vi "password.vi"() -> (0 "correct":bool)   [LabVIEW 2019]
uses:
  LLB/Commonly VI/Main Glb.vi
  <vilib>/Utility/xml.llb/Read From XML File(string).vi
  <vilib>/Utility/xml.llb/Write to XML File(string).vi
  Function/RobotCtrl Folder/Global/Robot_LinkData.vi
  LLB/Commonly VI.lvlib
panel:
  in  "Tab Control":enum32{"Page 1", "Page 2"}(tab)
  in  "1":bool
  in  "2":bool
  in  "3":bool
  in  "4":bool
  in  "5":bool
  in  "6":bool
  in  "7":bool
  in  "8":bool
  in  "9":bool
  in  "0":bool
  in  "String":string
  in  "check":bool
  in  "Cancel Button":bool
  in  "Seek Back Button":bool
  in  "Settings Button":bool
  in  "Stop Button":bool
  out "password":string
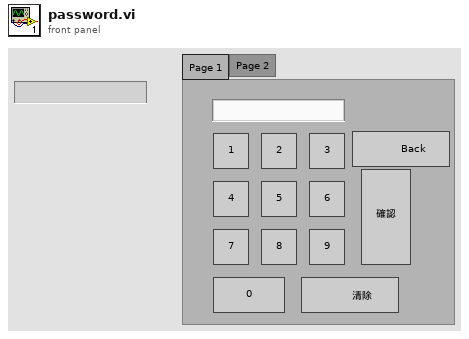
[diagram p1: front panel]
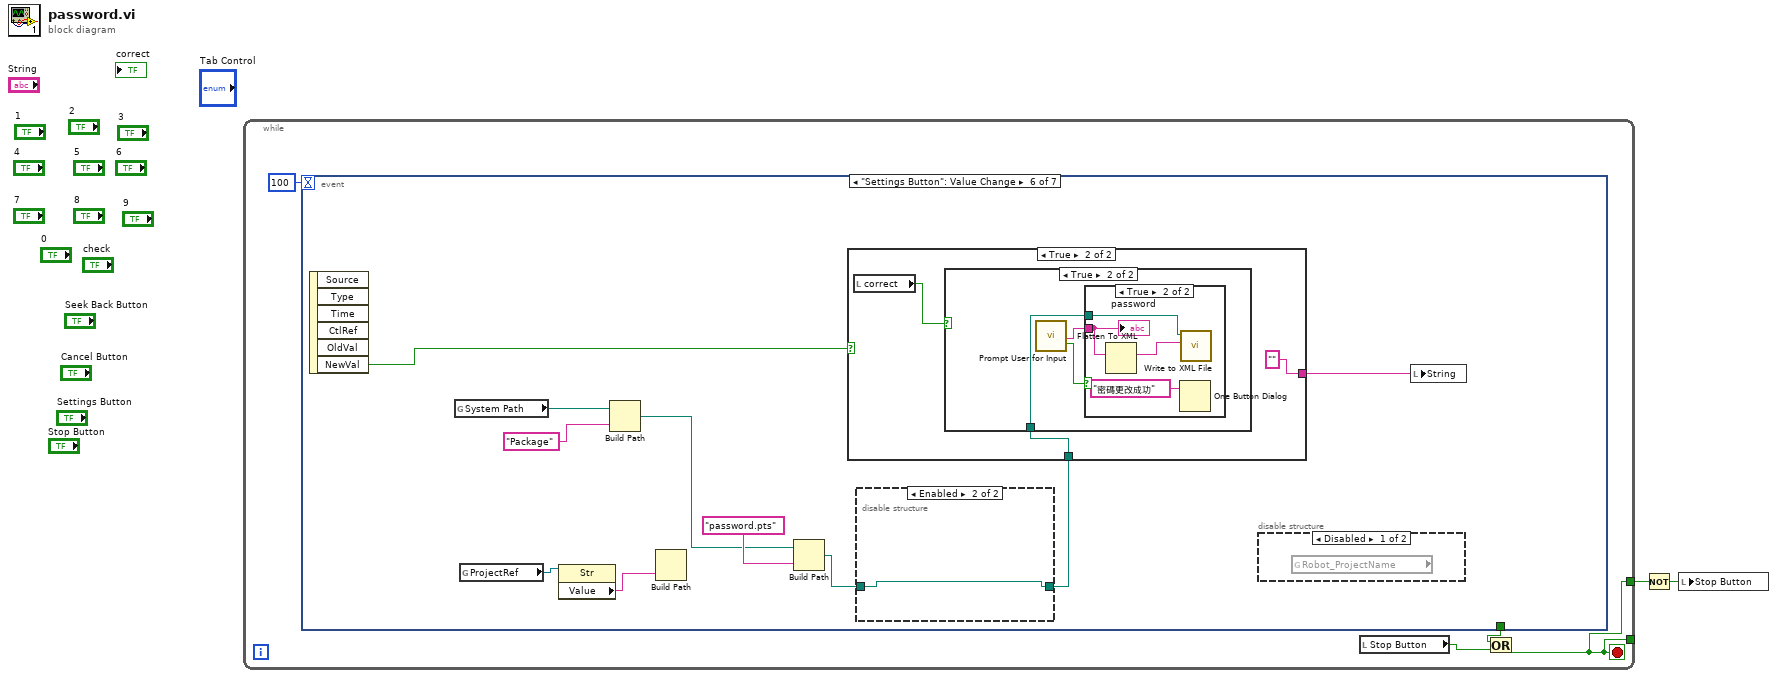
[diagram p0: block diagram]
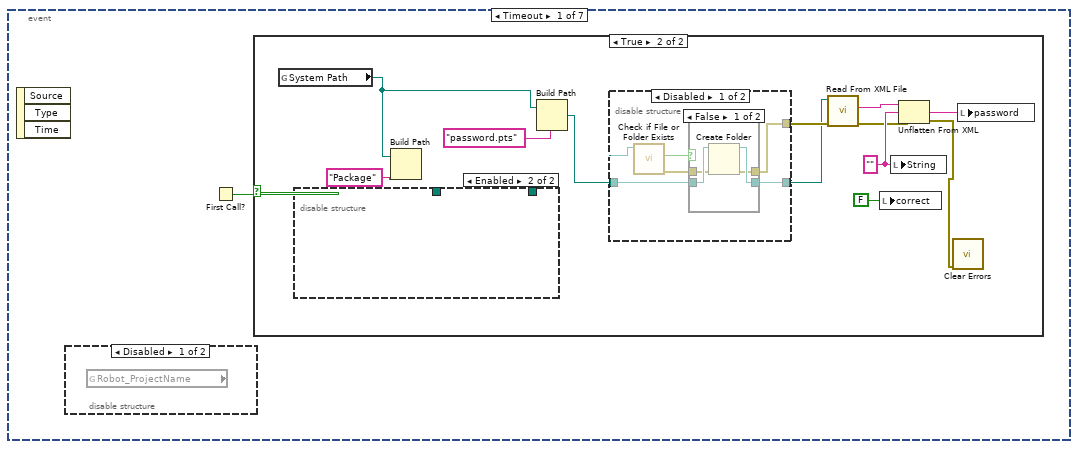
[diagram p2: hidden frame]
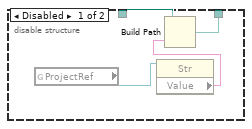
[diagram p7: hidden frame]
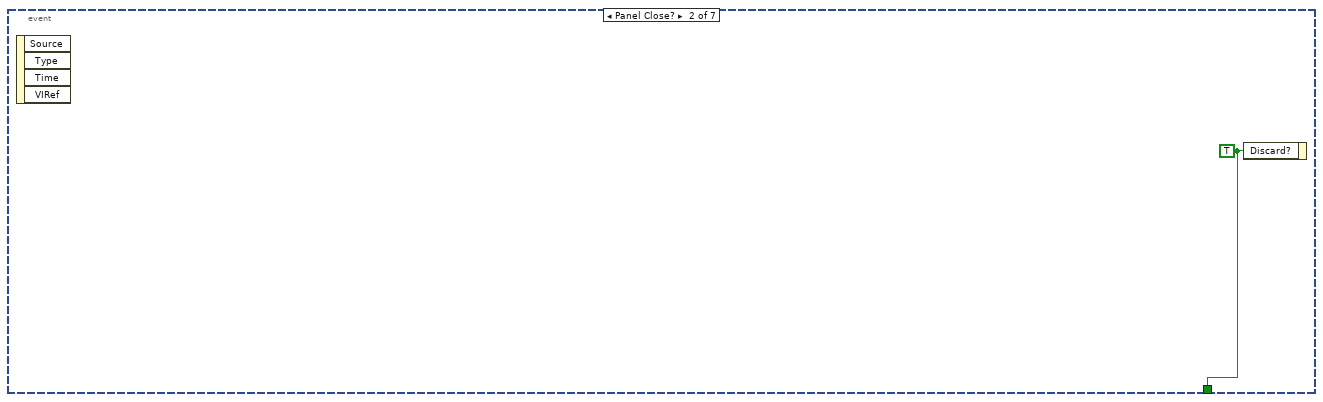
[diagram p8: hidden frame]
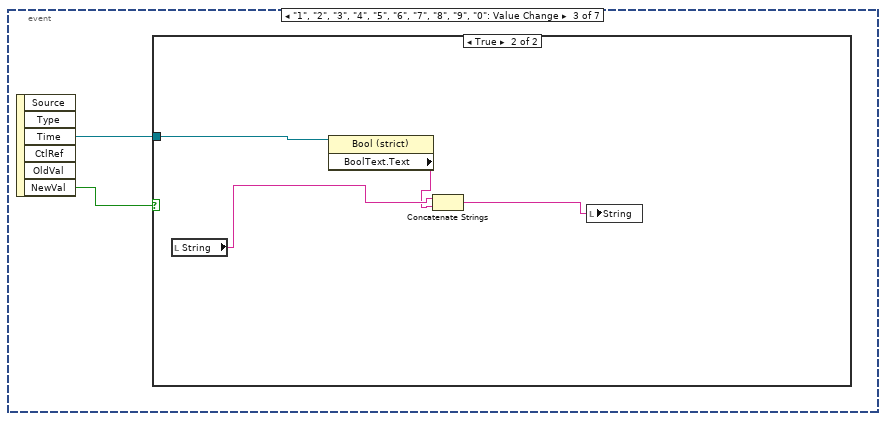
[diagram p9: hidden frame]
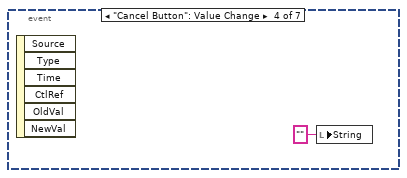
[diagram p11: hidden frame]
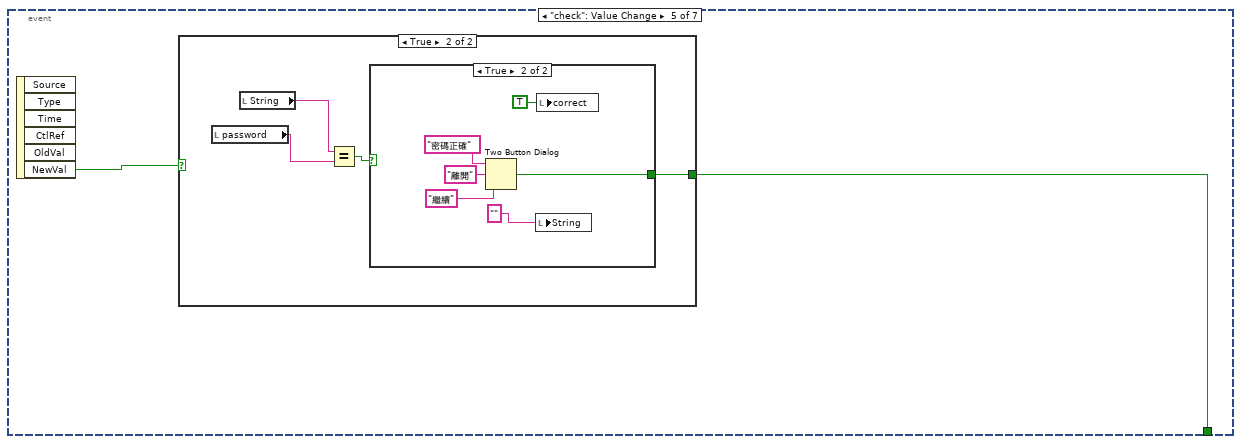
[diagram p12: hidden frame]
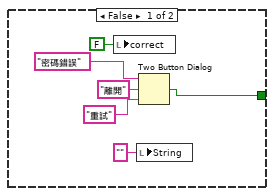
[diagram p14: hidden frame]
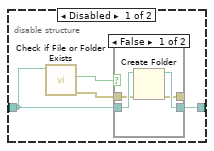
[diagram p15: hidden frame]
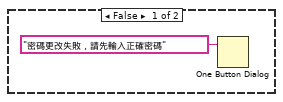
[diagram p19: hidden frame]
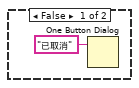
[diagram p20: hidden frame]
diagram:
  n1 = while {
    tunnel: [w3] -> _
    tunnel: [w3] -> w2
    stop <- w3 stop-if-true
    n2 = event shown="[5] \"Settings Button\": Value Change" {
      selector: _ -> [_ _ _ _ _ _ _]
      dyn-events: _ -> [_ _ _ _ _ _ _]
      timeout: 100 -> [_ _ _ _ _ _ _]
      tunnel: [_ w36 _ _ w44 _ _] -> w5
      event Timeout {
        n3 = event-data() -> ()  [unwired: 1 in, 3 out]
        n4 = disable-structure shown="Disabled" {
          frame Disabled {
            n5 = global read "Robot_LinkData.vi" "Robot_ProjectName"() -> ()  [unwired: 1 out]
          }
          frame Enabled {
          }
        }
        n6 = First Call?() -> (First Call?: T/F=w7:bool)
        n7 = case shown="True" w7 {
          frame False {
          }
          frame True {
            w17 = "" ("String")
            n8 = global read "Main Glb.vi" "System Path"() -> (w8:path)
            n9 = disable-structure shown="Enabled" {
              disable-tunnel: _ -> [w33 _]
              disable-tunnel: [w32 _] -> _
              frame Disabled {
                n10 = global read "Main Glb.vi" "ProjectRef"() -> (w34:refnum<vi>)
                n11 = property class="Str"(reference=w34) -> ("Value"=w35:string)  [unwired: 1 in, 2 out]
                n12 = Build Path(base path=w33, name or relative path=w35) -> (appended path=w32:path)
              }
              frame Enabled {
              }
            }
            n13 = Build Path(base path=w8, name or relative path="Package") -> ()  [unwired: 1 out]
            n14 = Build Path(base path=w8, name or relative path="password.pts") -> (appended path=w13:path)
            n15 = disable-structure shown="Disabled" {
              disable-tunnel: w13 -> [w22 w31]
              disable-tunnel: [w21 _] -> w12
              disable-tunnel: [w20 w31] -> w11
              frame Disabled {
                n16 = call <vilib>:"Check if File or Folder Exists.vi"("path"=w22) -> ("error out"=w23:errorcluster, "file or folder exists?"=w24:bool)  [unwired: 8 in, 1 out]
                n17 = case shown="False" w24 {
                  tunnel: w22 -> [w28 w30]
                  tunnel: [w27 w30] -> w20
                  tunnel: w23 -> [w26 w29]
                  tunnel: [w25 w29] -> w21
                  frame False {
                    n18 = Create Folder(path (use dialog)=w28, error in=w26) -> (created path=w27:path, error out=w25:errorcluster)  [unwired: 1 in, 1 out]
                  }
                  frame True {
                  }
                }
              }
              frame Enabled {
              }
            }
            n19 = call-poly <vilib>:"Read From XML File.vi"("error in (no error)"=w12, "XML File Path"=w11) -> ("error out"=w10:errorcluster, "XML Elements"=w18:string)  [unwired: 7 in, 1 out]
            n20 = local write "correct"(FALSE ("correct")) -> ()
            n21 = local write "String"(w17) -> ()
            n22 = Unflatten From XML(xml string=w18, type=w17, error in (no error)=w10) -> (value=w16:string, error out=w9:errorcluster)
            n23 = call <vilib>:"Clear Errors.vi"("error in (no error)"=w9) -> ()  [unwired: 5 in, 2 out]
            n24 = local write "password"(w16) -> ()
          }
        }
      }
      event Panel Close? {
        w36 = TRUE ("Discard?")
        n25 = event-data() -> ()  [unwired: 1 in, 4 out]
        n26 = event-data("Discard?"=w36) -> ()  [unwired: 1 in, 1 out]
      }
      event "1", "2", "3", "4", "5", "6", "7", "8", "9", "0": Value Change {
        n27 = event-data() -> ("CtlRef"=w38:refnum<vi>, "NewVal"=w37:bool)  [unwired: 1 in, 4 out]
        n28 = case shown="True" w37 {
          tunnel: w38 -> [_ w42]
          frame False {
          }
          frame True {
            n29 = local read "String"() -> (w41:string)
            n30 = property class="Bool (strict)"(reference=w42) -> ("BoolText.Text"=w40:string)  [unwired: 1 in, 2 out]
            n31 = Concatenate Strings(w41, w40) -> (w39:string)
            n32 = local write "String"(w39) -> ()
          }
        }
      }
      event "Cancel Button": Value Change {
        n33 = event-data() -> ()  [unwired: 1 in, 6 out]
        n34 = local write "String"("" ("String")) -> ()
      }
      event "check": Value Change {
        n35 = event-data() -> ("NewVal"=w45:bool)  [unwired: 1 in, 5 out]
        n36 = case shown="True" w45 {
          tunnel: [_ w46] -> w44
          frame False {
          }
          frame True {
            n37 = local read "password"() -> (w48:string)
            n38 = local read "String"() -> (w49:string)
            n39 = Equal?(x=w49, y=w48) -> (x = y?=w47:bool)
            n40 = case shown="True" w47 {
              tunnel: [w52 w58] -> w46
              frame False {
                n41 = local write "correct"(FALSE ("correct")) -> ()
                n42 = local write "String"("" ("String")) -> ()
                n43 = Two Button Dialog(message="密碼錯誤", 1:"重試" ("F button name (\"Cancel\")"), 2:"離開" ("T button name (\"OK\")")) -> (T button?=w52:bool)
              }
              frame True {
                n44 = Two Button Dialog(message="密碼正確", 1:"繼續" ("F button name (\"Cancel\")"), 2:"離開" ("T button name (\"OK\")")) -> (T button?=w58:bool)
                n45 = local write "String"("" ("String")) -> ()
                n46 = local write "correct"(TRUE ("correct")) -> ()
              }
            }
          }
        }
      }
      event "Settings Button": Value Change {
        n47 = event-data() -> ("NewVal"=w71:bool)  [unwired: 1 in, 5 out]
        n48 = global read "Main Glb.vi" "System Path"() -> (w66:path)
        n49 = global read "Main Glb.vi" "ProjectRef"() -> (w63:refnum<vi>)
        n50 = property class="Str"(reference=w63) -> ("Value"=w67:string)  [unwired: 1 in, 2 out]
        n51 = Build Path(base path=w66, name or relative path="Package") -> (appended path=w62:path)
        n52 = Build Path(name or relative path=w67) -> ()  [unwired: 1 in, 1 out]
        n53 = Build Path(base path=w62, name or relative path="password.pts") -> (appended path=w65:path)
        n54 = disable-structure shown="Enabled" {
          disable-tunnel: w65 -> [w73 w82]
          disable-tunnel: [w72 w82] -> w64
          frame Disabled {
            n55 = call <vilib>:"Check if File or Folder Exists.vi"("path"=w73) -> ("error out"=w75:errorcluster, "file or folder exists?"=w74:bool)  [unwired: 8 in, 1 out]
            n56 = case shown="False" w74 {
              tunnel: w73 -> [w79 w81]
              tunnel: [w78 w81] -> w72
              tunnel: w75 -> [w77 w80]
              tunnel: [w76 w80] -> _
              frame False {
                n57 = Create Folder(path (use dialog)=w79, error in=w77) -> (created path=w78:path, error out=w76:errorcluster)  [unwired: 1 in, 1 out]
              }
              frame True {
              }
            }
          }
          frame Enabled {
          }
        }
        n58 = case shown="True" w71 {
          tunnel: [_ "" ("String")] -> w70
          tunnel: w64 -> [_ w83]
          frame False {
          }
          frame True {
            n59 = local read "correct"() -> (w85:bool)
            n60 = case shown="True" w85 {
              tunnel: w83 -> [_ w87]
              frame False {
                n61 = One Button Dialog(message="密碼更改失敗，請先輸入正確密碼") -> ()  [unwired: 1 in, 1 out]
              }
              frame True {
                n62 = call "Prompt User for Input"() -> ("Password"=w88:string, "OK"=w89:bool)  [unwired: 17 in, 1 out]
                n63 = case shown="True" w89 {
                  tunnel: w88 -> [_ w92]
                  tunnel: w87 -> [_ w91]
                  frame False {
                    n64 = One Button Dialog(message="已取消") -> ()  [unwired: 1 in, 1 out]
                  }
                  frame True {
                    n65 = Flatten To XML(anything=w92) -> (xml string=w93:string)
                    n66 = One Button Dialog(message="密碼更改成功") -> ()  [unwired: 1 in, 1 out]
                    n67 = call-poly <vilib>:"Write to XML File.vi"("XML Input"=w93, "XML File Path"=w91) -> ()  [unwired: 7 in, 3 out]
                    "password" <- w92
                  }
                }
              }
            }
          }
        }
        n68 = disable-structure shown="Disabled" {
          frame Disabled {
            n69 = global read "Robot_LinkData.vi" "Robot_ProjectName"() -> ()  [unwired: 1 out]
          }
          frame Enabled {
          }
        }
        n70 = local write "String"(w70) -> ()
      }
      event "Seek Back Button": Value Change {
        n71 = event-data() -> ("NewVal"=w96:bool)  [unwired: 1 in, 5 out]
        n72 = local read "String"() -> (w95:string)
        n73 = case shown="True" w96 {
          tunnel: w95 -> [_ w101]
          tunnel: w95 -> [_ w99]
          frame False {
          }
          frame True {
            n74 = String Length(string=w101) -> (length=w98:i32)
            n75 = Decrement(x=w98) -> (x-1=w97:i32)
            n76 = String Subset(string=w99, length (rest)=w97) -> (substring=w100:string)  [unwired: 1 in]
            n77 = local write "String"(w100) -> ()
          }
        }
      }
    }
    n78 = local read "Stop Button"() -> (w4:bool)
    n79 = Or(x=w5, y=w4) -> (x .or. y?=w3:bool)
  }
  n80 = Not(x=w2) -> (.not. x?=w1:bool)
  n81 = local write "Stop Button"(w1) -> ()
